vi "Overlay Offset Centroids.vi"(9 "Bounding Rect":T3, 10 "Particle Reports (Pixels)":T2(array[cluster]), 11 "Image":T1) -> (3 "Image Out":T1)   [LabVIEW 2011]
uses:
  <vilib>/vision/Image Controls.llb/IMAQ Image.ctl
  <vilib>/vision/NI_Vision_Development_Module.lvlib
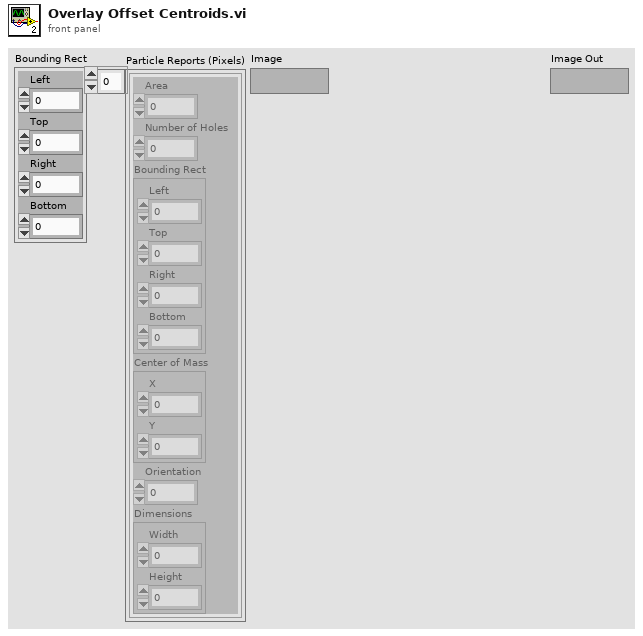
[diagram p1: front panel]
types:
  T1 = typedef "IMAQ Image.ctl" = refnum<image>
  T2 = cluster{"Area":dbl, "Number of Holes":dbl, "Bounding Rect":cluster{"Left":dbl, "Top":dbl, "Right":dbl, "Bottom":dbl}, "Center of Mass":cluster{"X":dbl, "Y":dbl}, "Orientation":dbl, "Dimensions":cluster{"Width":dbl, "Height":dbl}}[]
  T3 = cluster{"Left":dbl, "Top":dbl, "Right":dbl, "Bottom":dbl}
  T4 = typedef "Image Type" = u32
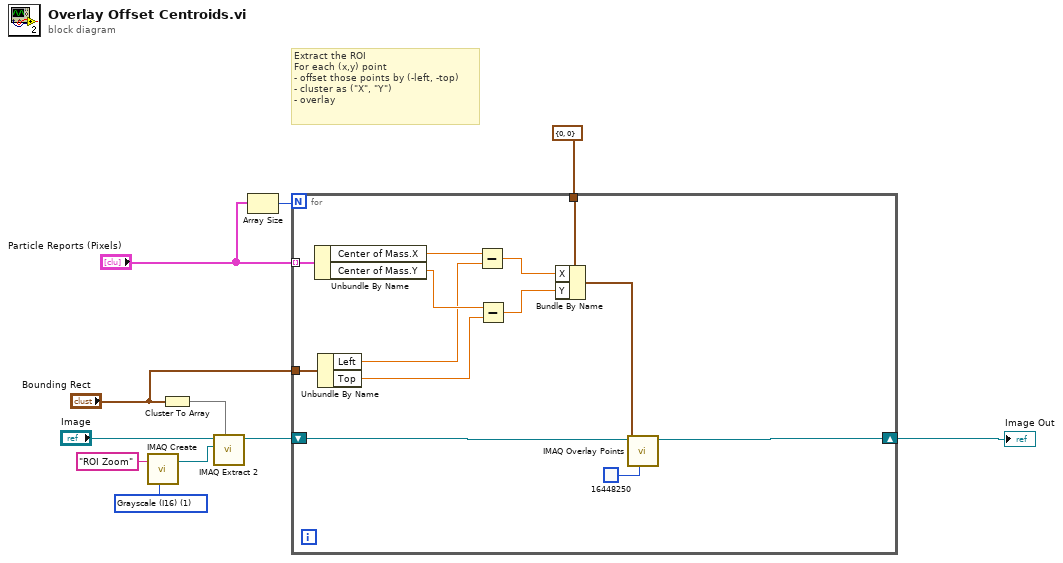
[diagram p0: block diagram]
diagram:
  w2 = T4 1 items=["Grayscale (U8)", "Grayscale (I16)", "Grayscale (SGL)", "Complex (CSG)", "RGB (U32)", "HSL (U32)", "RGB (U64)", "Grayscale (U16)"] ("Image Type")
  # "Extract the ROI\nFor each (x,y) point\n- offset those points by (-left, -top)\n- cluster as (\"X\", \"Y\")\n- overlay"
  n1 = call "IMAQ Create"("Image Name"="ROI Zoom", "Image Type"=w2) -> ("New Image"=w3:T1)  [unwired: 3 in, 1 out]
  n2 = Cluster To Array(cluster="Bounding Rect") -> (array=w7:dbl[])
  n3 = call "IMAQ Extract 2"("Optional Rectangle"=w7, "Image Dst"=w3, "Image Src"="Image") -> ("Image Dst Out"=w5:T1)  [unwired: 7 in, 1 out]
  n4 = Array Size(array="Particle Reports (Pixels)") -> (size(s)=w11:i32)
  n5 = for {
    N: w11 -> [_]
    tunnel: "Particle Reports (Pixels)" -> [w24] mode=indexing
    tunnel: cluster{"X":i32, "Y":i32} {"X"=0, "Y"=0} -> [w21]
    tunnel: "Bounding Rect" -> [w17]
    shift-right: [w13] -> w4
    shift-left: w5 -> [w14]
    n6 = Unbundle By Name(w24) -> ("Center of Mass.X"=w23:dbl, "Center of Mass.Y"=w22:dbl)
    n7 = Unbundle By Name(w17) -> ("Left"=w16:dbl, "Top"=w15:dbl)
    n8 = Subtract(x=w23, y=w16) -> (x-y=w20:dbl)
    n9 = Subtract(x=w22, y=w15) -> (x-y=w19:dbl)
    n10 = Bundle By Name(cluster=w21, "X"=w20, "Y"=w19) -> (w18:cluster{"X":i32, "Y":i32})
    n11 = call "IMAQ Overlay Points"("Color"=u32 16448250, "Point"=w18, "Image"=w14) -> ("Image Out"=w13:T1)  [unwired: 7 in, 1 out]
  }
  "Image Out" <- w4
